vi "Inspect.vi"(9 "From Msg Event":bool, 10 "Msg in":refnum<class "Msg.lvclass">, 11 "Core Actor in":refnum<class "Core Actor.lvclass">) -> (2 "Msg out":refnum<class "Msg.lvclass">, 3 "Core Actor out":refnum<class "Core Actor.lvclass">)   [LabVIEW 2025, in "jettl.lvlib" / "Actor.lvlib" / "Core Actor.lvclass"]
uses:
  Core Actor.lvclass
  Msg/Msg.lvclass
  Core Actor.lvclass/Core Actor.ctl
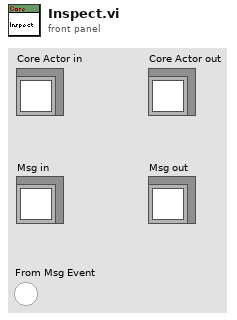
[diagram p1: front panel]
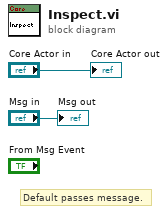
[diagram p0: block diagram]
diagram:
  # "Default passes message."
  "Core Actor out" <- "Core Actor in"
  "Msg out" <- "Msg in"
